vi "Power整体图.vi"() -> ()   [LabVIEW 2014]
panel:
  in  "Energy":bool
  in  "Emit":bool
  in  "Disconnect":bool
  in  "Connect":bool
  in  "Charge":bool
  in  "Cache":bool
  in  "Power":bool
  in  "No emit":bool
  in  "No charge":bool
  in  "No battery":bool
  in  "Flash":bool
  in  "Established":bool
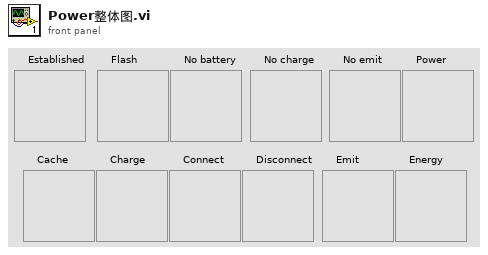
[diagram p1: front panel]
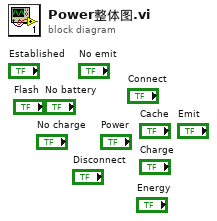
[diagram p0: block diagram]
diagram:
